vi "Array - Not Equivalent.vi"() -> ()   [LabVIEW 2017, in "Assertions.Tests.lvlib" / "Assert Collection Equivalent.lvlib"]
uses:
  Assert Collection Equivalent.lvlib
  d2c6a248-d56f-4fec-a1e4-367730173575.vi
  src/Transparent Assertions/Constraints/Collection Is Equivalent/Create.vi
  src/Transparent Assertions/Constraints/Collection Is Equivalent/Collection Is Equivalent.lvclass
  src/Transparent Assertions/Assertions/Assertions.lvlib
panel:
  out "error out":errorcluster
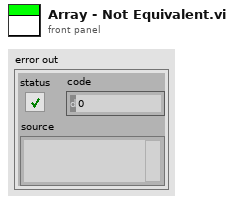
[diagram p1: front panel]
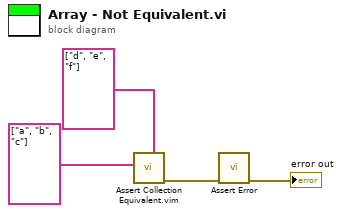
[diagram p0: block diagram]
diagram:
  n1 = call "Assert Collection Equivalent.vim"("Expected"=string[] ["d", "e", "f"], "Collection"=string[] ["a", "b", "c"]) -> ("error out"=w2:errorcluster)  [unwired: 9 in]
  n2 = call "Assert Error.vi"("error in (no error)"=w2) -> ("error out"=→"error out":errorcluster)  [unwired: 10 in]
